vi "USB relay.vi"(10 "Relay on":bool, 11 "USB relay com port":refnum<visa-resource-name>="COM5") -> (2 "read buffer":string)   [LabVIEW 2015]
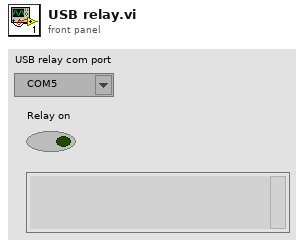
[diagram p1: front panel]
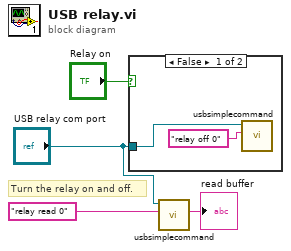
[diagram p0: block diagram]
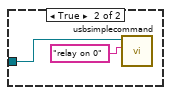
[diagram p2: hidden frame]
diagram:
  # "Turn the relay on and off."
  n1 = case shown="False" "Relay on" {
    tunnel: "USB relay com port" -> [w6 w8]
    frame False {
      n2 = call "usbsimplecommand.vi"("write buffer"="relay off 0", "VISA resource name"=w6) -> ()  [unwired: 9 in, 1 out]
    }
    frame True {
      n3 = call "usbsimplecommand.vi"("write buffer"="relay on 0", "VISA resource name"=w8) -> ()  [unwired: 9 in, 1 out]
    }
  }
  n4 = call "usbsimplecommand.vi"("write buffer"="relay read 0", "VISA resource name"="USB relay com port") -> ("read buffer"=→"read buffer":string)  [unwired: 9 in]
